vi "_Unlock CSMQ.vi"(8 "Error in":errorcluster caption="Error in (no error)", 11 "CSMQ in":T1) -> (0 "Error out":errorcluster, 3 "CSMQ out":T1)   [LabVIEW 2014, in "Communicable State Machine.lvlib"]
uses:
  Communicable State Machine.lvlib
  _CSMQ.ctl
  Typedef/_Cross JKISM State Response.ctl
  Typedef/_Cross JKISM State Data.ctl
  Typedef/_CSM_MSG_TYPE.ctl
  Typedef/_CSM_MODE.ctl
  Typedef/_CSM Status Change Event Data.ctl
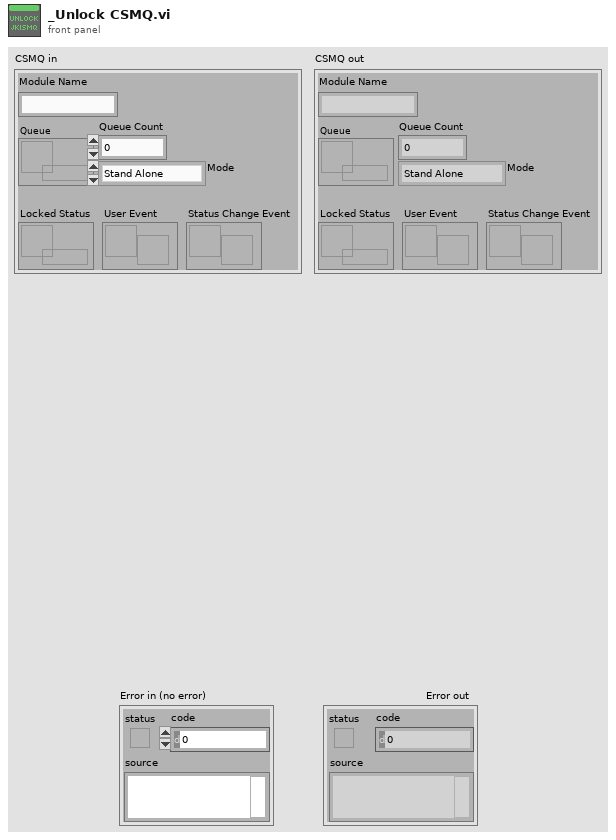
[diagram p1: front panel]
types:
  T1 = typedef "Communicable State Machine.lvlib/_CSMQ.ctl" = cluster{"Module Name":string, "Queue":refnum<queue>, "Locked Status":refnum<data-value>, "Mode":T2, "User Event":refnum<user-event>, "Queue Count":i32, "Status Change Event":refnum<user-event>}
  T2 = typedef "Communicable State Machine.lvlib/_CSM_MODE.ctl" = enum16{"Stand Alone", "JKISM", "Action Worker"}
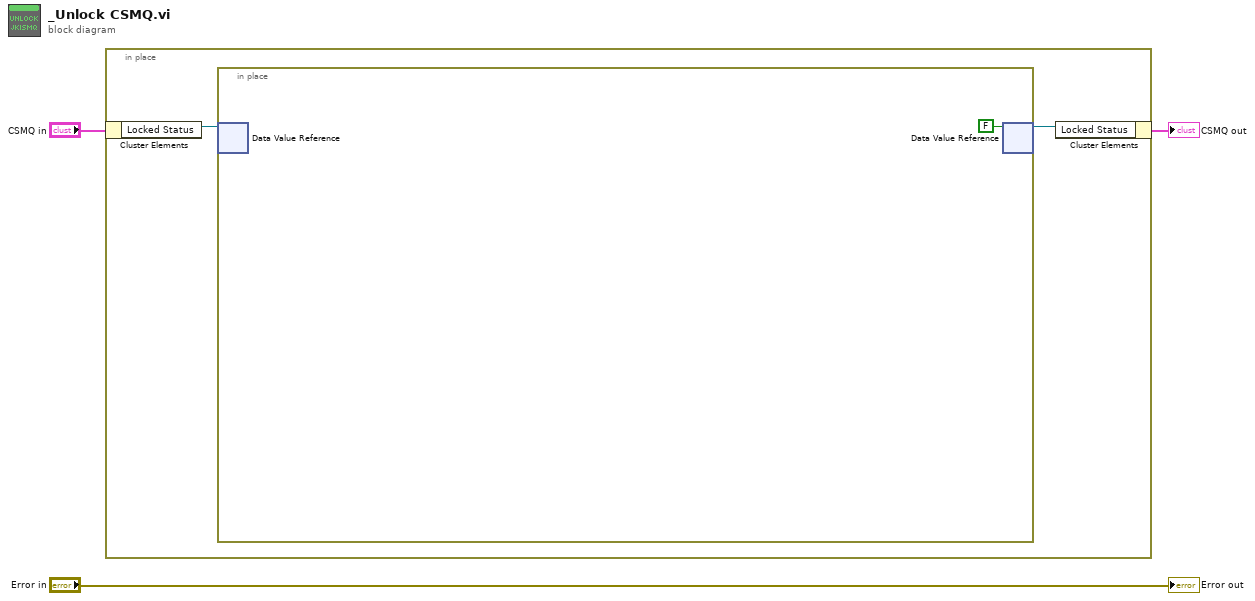
[diagram p0: block diagram]
diagram:
  n1 = in-place "In Place Element Structure" {
    n2 = in-place-cluster #1("CSMQ in") -> ("Locked Status"=w5:refnum<data-value>)
    n3 = in-place {
      n4 = in-place-dvr #2(w5) -> ()  [unwired: 2 out]
      n5 = in-place-dvr #2(FALSE ("data value")) -> (w4:refnum<data-value>)  [unwired: 1 out]
    }
    n6 = in-place-cluster #1("Locked Status"=w4) -> (→"CSMQ out":T1)
  }
  "Error out" <- "Error in"
